vi "Receive.vi"(8 "error in (no error)":errorcluster, 9 "timeout in ms (0)":i32, 11 "Network_Streams in":T1) -> (0 "error out":errorcluster, 1 "Timeout?":bool, 2 "Packet Data":u8[](array[numeric]), 3 "Network_Streams out":T1)   [LabVIEW 2020, in "Communication VIs.lvlib" / "Network.lvlib"]
uses:
  Network.lvlib
  Network Streams.ctl
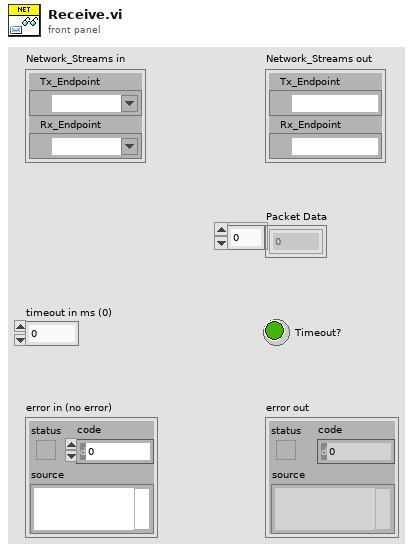
[diagram p1: front panel]
types:
  T1 = typedef "Communication VIs.lvlib/Network.lvlib/Network Streams.ctl" = cluster{"Tx_Endpoint":refnum<k21>, "Rx_Endpoint":refnum<k21>}
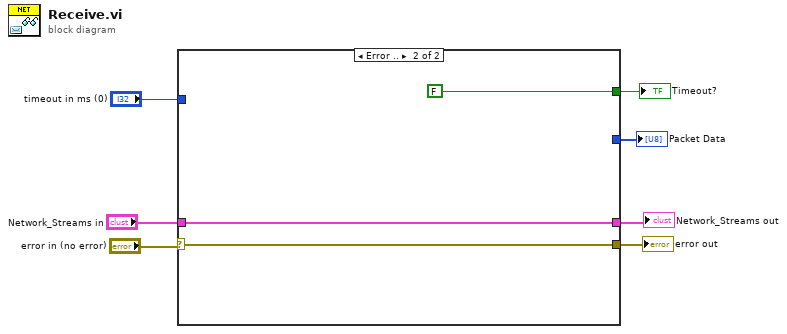
[diagram p0: block diagram]
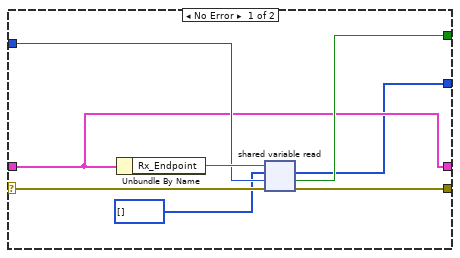
[diagram p2: hidden frame]
diagram:
  n1 = case shown="Error .." "error in (no error)" {
    selector: "error in (no error)" -> [w12 w17]
    tunnel: "timeout in ms (0)" -> [w13 _]
    tunnel: [w11 w17] -> w5
    tunnel: [w14 FALSE ("timed out?")] -> w4
    tunnel: "Network_Streams in" -> [w9 w16]
    tunnel: [w9 w16] -> w2
    tunnel: [w8 _] -> w1
    frame No Error {
      n2 = Unbundle By Name(w9) -> ("Rx_Endpoint"=w15:refnum<k21>)
      n3 = shared-variable-read(w15, w12, u8[] [], w13) -> (w11:errorcluster, w14:bool, w8:u8[])  [unwired: 1 out]
    }
    frame Error {
    }
  }
  "error out" <- w5
  "Timeout?" <- w4
  "Network_Streams out" <- w2
  "Packet Data" <- w1
